vi "ResultDialog.vi"(8 "error in (no error)":errorcluster, 10 "Result Array":string[](array[string])) -> (0 "error out":errorcluster)   [LabVIEW 2015]
uses:
  V:/SepOfConcerns/Source/DotNet/ClientDialogs/ClientDialogs/bin/Debug/ClientDialogs.dll
  DotNet/ClientDialogs/ClientDialogs/bin/Debug/ClientDialogs.dll
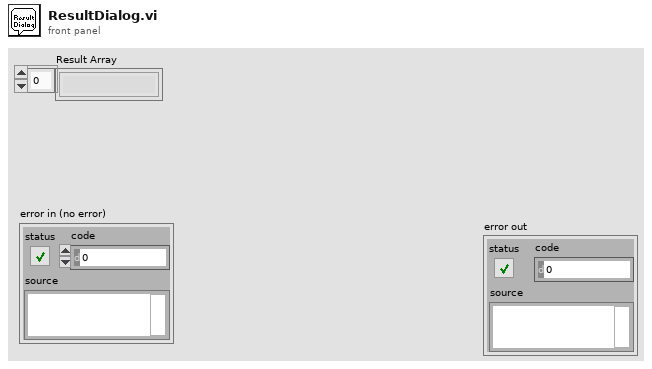
[diagram p1: front panel]
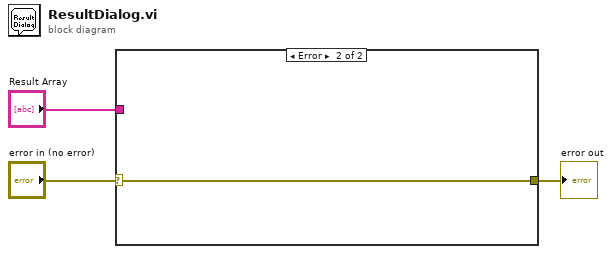
[diagram p0: block diagram]
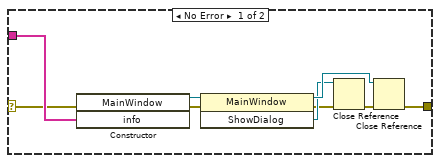
[diagram p2: hidden frame]
diagram:
  n1 = case shown="Error" "error in (no error)" {
    selector: "error in (no error)" -> [w4 w13]
    tunnel: "Result Array" -> [w12 _]
    tunnel: [w8 w13] -> w2
    frame No Error {
      n2 = constructor class="MainWindow"(error in=w4, "info"=w12) -> (reference out=w11:refnum<k24>, error out=w9:errorcluster)  [unwired: 2 in, 2 out]
      n3 = invoke class="MainWindow" method="ShowDialog"(reference=w11, error in=w9) -> (reference out=w10:refnum<k24>, error out=w6:errorcluster, "ShowDialog"=w7:refnum<k24>)  [unwired: 1 in]
      n4 = Close Reference(reference=w7, error in (no error)=w6) -> (error out=w5:errorcluster)
      n5 = Close Reference(reference=w10, error in (no error)=w5) -> (error out=w8:errorcluster)
    }
    frame Error {
    }
  }
  "error out" <- w2
